vi "motor encoder.vi"(8 "Error In":errorcluster, 9 "Motor Reset":bool, 10 "Motor Enum":T1, 11 "FPGA VI Reference In":refnum<k20>) -> (0 "Error Out":errorcluster, 1 "encoder out":i32, 3 "FPGA VI Reference Out":refnum<k20>)   [LabVIEW 2019, in "Motor single.lvclass"]
uses:
  Motor single.lvclass
  motor enum(FPGA).ctl
  <vilib>/Utility/error.llb/Error Cluster From Error Code.vi
  <vilib>/rvi/errors/niLvFpgaAdjustHostInterfaceError.vi
  <vilib>/rvi/interface/nirviReadWriteControl/nirviReadWriteControl.xnode
  NiFpgaLv.dll
  <vilib>/rvi/interface/Simulation/niFpgaSimulationCallBeginRW.vi
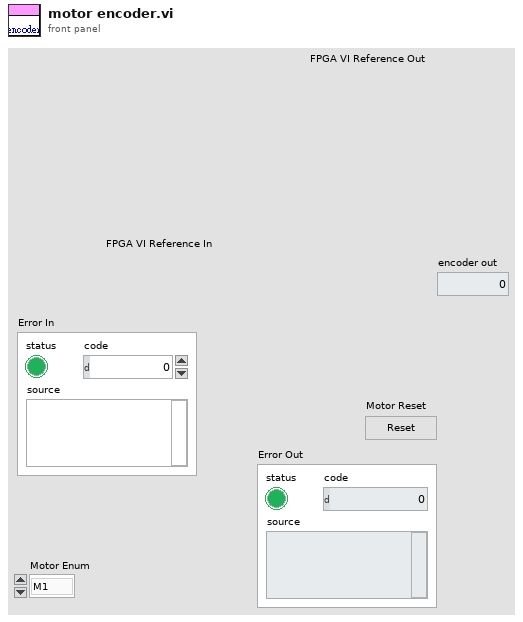
[diagram p1: front panel]
types:
  T1 = typedef "Motor single.lvclass/motor enum(FPGA).ctl" = enum16{"M1", "M2", "M3", "M4"}
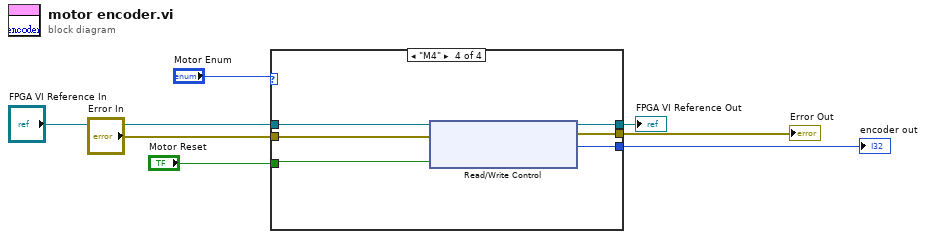
[diagram p0: block diagram]
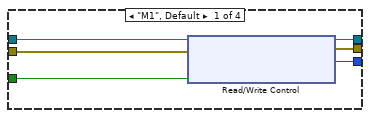
[diagram p2: hidden frame]
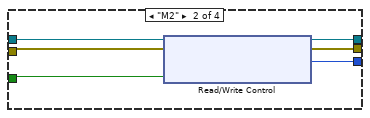
[diagram p3: hidden frame]
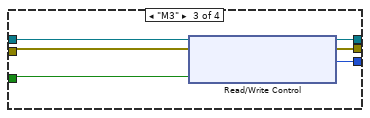
[diagram p4: hidden frame]
diagram:
  n1 = case shown="\"M4\"" "Motor Enum" {
    tunnel: "FPGA VI Reference In" -> [w13 w19 w25 w30]
    tunnel: "Error In" -> [w12 w18 w24 w29]
    tunnel: "Motor Reset" -> [w11 w17 w23 w31]
    tunnel: [w8 w16 w22 w28] -> w1
    tunnel: [w10 w15 w21 w27] -> w3
    tunnel: [w9 w14 w20 w26] -> w2
    frame "M1", Default {
      n2 = xnode "Read/Write Control"("FPGA VI Reference In"=w13, "error in"=w12, "Motor1.encoder_Reset"=w11) -> ("FPGA VI Reference Out"=w9:refnum<k20>, "error out"=w10:errorcluster, "Motor1.encoder"=w8:i32)
    }
    frame "M2" {
      n3 = xnode "Read/Write Control"("FPGA VI Reference In"=w19, "error in"=w18, "Motor2.encoder_Reset"=w17) -> ("FPGA VI Reference Out"=w14:refnum<k20>, "error out"=w15:errorcluster, "Motor2.encoder"=w16:i32)
    }
    frame "M3" {
      n4 = xnode "Read/Write Control"("FPGA VI Reference In"=w25, "error in"=w24, "Motor3.encoder_Reset"=w23) -> ("FPGA VI Reference Out"=w20:refnum<k20>, "error out"=w21:errorcluster, "Motor3.encoder"=w22:i32)
    }
    frame "M4" {
      n5 = xnode "Read/Write Control"("FPGA VI Reference In"=w30, "error in"=w29, "Motor4.encoder_Reset"=w31) -> ("FPGA VI Reference Out"=w26:refnum<k20>, "error out"=w27:errorcluster, "Motor4.encoder"=w28:i32)
    }
  }
  "Error Out" <- w3
  "FPGA VI Reference Out" <- w2
  "encoder out" <- w1
